vi "replaceAmountToken.vi"(8 "error in (no error)":errorcluster, 10 "Query In":string, 11 "Transaction in":refnum<class "Transaction.lvclass">) -> (0 "error out":errorcluster, 2 "Query Out":string, 3 "Transaction out":refnum<class "Transaction.lvclass">)   [LabVIEW 2018, in "Transaction.lvclass"]
uses:
  Transaction.lvclass
  Transaction.lvclass/Transaction.ctl
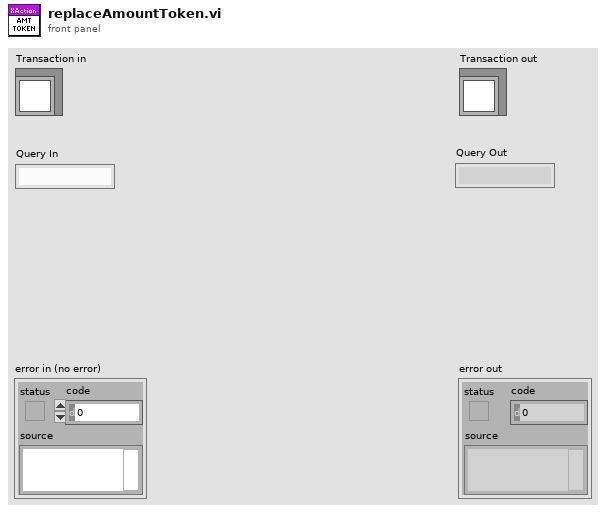
[diagram p1: front panel]
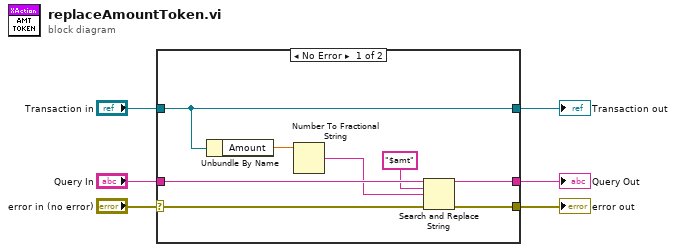
[diagram p0: block diagram]
diagram:
  n1 = case shown="No Error" "error in (no error)" {
    selector: "error in (no error)" -> [w13 w17]
    tunnel: [w12 w17] -> w5
    tunnel: [w14 w16] -> w3
    tunnel: "Transaction in" -> [w14 w16]
    tunnel: "Query In" -> [w11 w15]
    tunnel: [w10 w15] -> w1
    frame No Error {
      n2 = Unbundle By Name(w14) -> ("Amount"=w9:dbl)
      n3 = Number To Fractional String(number=w9) -> (F-format string=w8:string)  [unwired: 3 in]
      n4 = Search and Replace String(input string=w11, search string="$amt", replace string=w8, error in=w13) -> (result string=w10:string, error out=w12:errorcluster)  [unwired: 4 in, 2 out]
    }
    frame Error {
    }
  }
  "error out" <- w5
  "Transaction out" <- w3
  "Query Out" <- w1
